vi "v0.2_limpiar_encoder_serial.vi"(8 "error in (no error)":errorcluster, 11 "VISA COM IN":refnum<visa-resource-name>) -> (0 "error out":errorcluster, 3 "VISA COM OUT":refnum<visa-resource-name>)   [LabVIEW 2011]
doc: "<B>PTO Salida de tren de pulsos</B>\n\nCambiar la frecuencia de salida. Un valor de cero detiene el motor. Existe un valor máximo luego del cual el servomotor se detiene, este valor depende de los paràmetros del driver.\n<B>Frecuencia </B> Valor en hertzios del tren de pulsos a la salida del microcontrolador mbed."
panel:
  # "Encerar el contador del encoder"
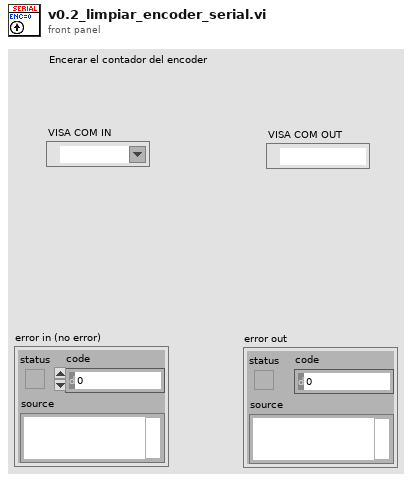
[diagram p1: front panel]
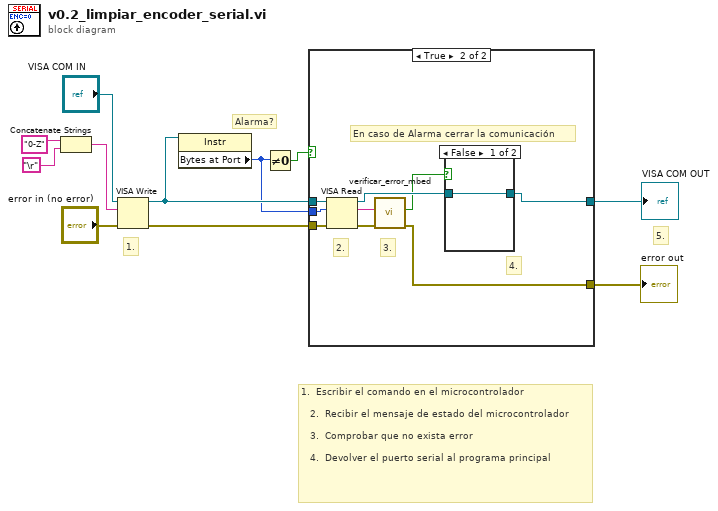
[diagram p0: block diagram]
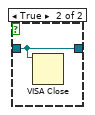
[diagram p3: hidden frame]
diagram:
  # "1.  Escribir el comando en el microcontrolador   \n\n   2.  Recibir el mensaje de estado del microcontrolador   \n\n   3.  Comprobar que no exista error\n\n   4.  Devolver el puerto serial al programa principal"
  # "5."
  # "1."
  # "3."
  # "2."
  # "4."
  # "Alarma?"
  n1 = Concatenate Strings("0-Z" ("string"), "\r") -> (w10:string)
  n2 = VISA Write(VISA resource name="VISA COM IN", write buffer=w10, error in (no error)="error in (no error)") -> (VISA resource name out=w5:refnum<visa-resource-name>, error out=w7:errorcluster)  [unwired: 1 out]
  n3 = property class="Instr"(reference=w5) -> ("Bytes at Port"=w3:u32)  [unwired: 1 in, 2 out]
  n4 = Not Equal To 0?(x=w3) -> (x != 0?=w4:bool)
  n5 = case shown="True" w4 {
    tunnel: w5 -> [w13 w19]
    tunnel: w7 -> [w12 w18]
    tunnel: w3 -> [_ w16]
    tunnel: [w13 w15] -> w2
    tunnel: [w12 w14] -> w1
    frame False {
    }
    frame True {
      # "En caso de Alarma cerrar la comunicación"
      n6 = VISA Read(VISA resource name=w19, byte count=w16, error in (no error)=w18) -> (VISA resource name out=w20:refnum<visa-resource-name>, read buffer=w21:string, error out=w22:errorcluster)  [unwired: 1 out]
      n7 = call "verificar_error_mbed.vi"("error in (no error)"=w22, "desde_mbed"=w21) -> ("error out"=w14:errorcluster, "error?"=w17:bool)  [unwired: 8 in]
      n8 = case shown="False" w17 {
        tunnel: w20 -> [w23 w24]
        tunnel: [w23 w24] -> w15
        frame False {
        }
        frame True {
          n9 = VISA Close(VISA resource name=w24) -> ()  [unwired: 1 in, 1 out]
        }
      }
    }
  }
  "VISA COM OUT" <- w2
  "error out" <- w1
